vi "save_variables_table.vi"(8 "error in":errorcluster, 10 "Variable Settings.Variables":T1(array[cluster]), 11 "base path":path) -> (0 "error out":errorcluster)   [LabVIEW 2013]
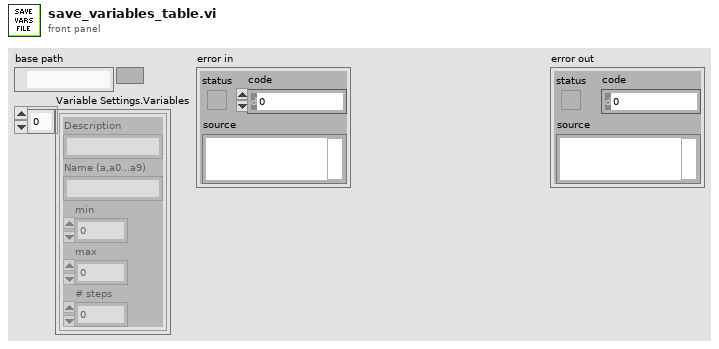
[diagram p1: front panel]
types:
  T1 = cluster{"Description":string, "Name (a,a0...a9)":string, "min":dbl, "max":dbl, "# steps":u32}[]
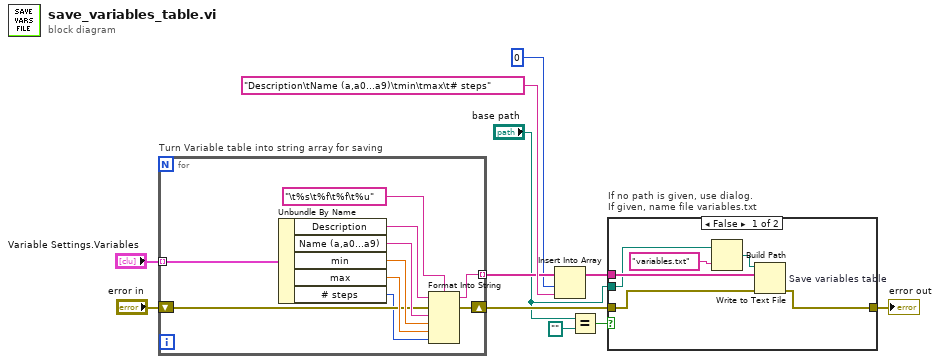
[diagram p0: block diagram]
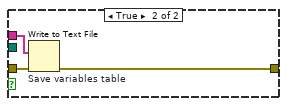
[diagram p2: hidden frame]
diagram:
  n1 = for "Turn Variable table into string array for saving" {
    tunnel: "Variable Settings.Variables" -> [w12] mode=indexing
    shift-right: [w15] -> w6
    shift-left: "error in" -> [w16]
    tunnel: [w14] -> w8 mode=indexing
    n2 = Unbundle By Name(w12) -> ("Description"=w20:string, "Name (a,a0...a9)"=w19:string, "min"=w18:dbl, "max"=w17:dbl, "# steps"=w13:u32)
    n3 = Format Into String(format string="\t%s\t%f\t%f\t%u", initial string=w20, error in=w16, w19, w18, w17, w13) -> (resulting string=w14:string, error out=w15:errorcluster)
  }
  n4 = Insert Into Array(array=w8, index=0, new element="Description\tName (a,a0...a9)\tmin\tmax\t# steps" ("new element/subarray")) -> (w2:string[])
  n5 = Equal?(x="base path", y=path "") -> (x = y?=w3:bool)
  n6 = case "If no path is given, use dialog.\nIf given, name file variables.txt" shown="False" w3 {
    tunnel: w6 -> [w23 w30]
    tunnel: [w22 w29] -> w5
    tunnel: w2 -> [w27 w28]
    tunnel: "base path" -> [w24 _]
    frame False {
      n7 = Build Path(base path=w24, name or relative path="variables.txt") -> (appended path=w25:path)
      n8 = Write to Text File "Save variables table"(file (use dialog)=w25, text=w27, error in=w23) -> (error out=w22:errorcluster)  [unwired: 1 in, 2 out]
    }
    frame True {
      n9 = Write to Text File "Save variables table"(text=w28, error in=w30) -> (error out=w29:errorcluster)  [unwired: 2 in, 2 out]
    }
  }
  "error out" <- w5
